vi "indexOf.vi"(8 "error in (no error)":errorcluster, 10 "Key":string, 11 "Bucket in":refnum<class "Bucket.lvclass">) -> (0 "error out":errorcluster, 2 "Index":i32, 3 "Bucket out":refnum<class "Bucket.lvclass">)   [LabVIEW 2017, in "Bucket.lvclass"]
uses:
  <userlib>/836-Library/Data_Structures/HashMap/Support/Bucket/Bucket.lvclass
  <userlib>/836-Library/Data_Structures/HashMap/Support/Bucket/Bucket.lvclass/Bucket.ctl
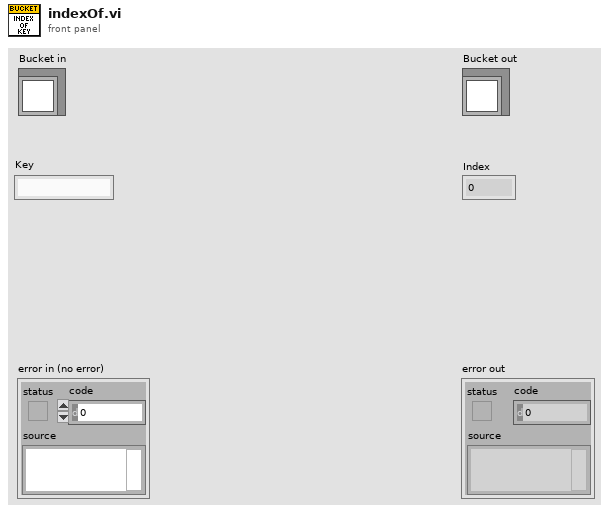
[diagram p1: front panel]
types:
  T1 = typedef "KeyValuePair.ctl" = cluster{"Key":string, "Value":variant}
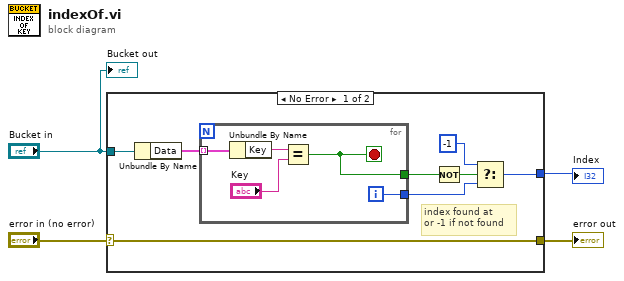
[diagram p0: block diagram]
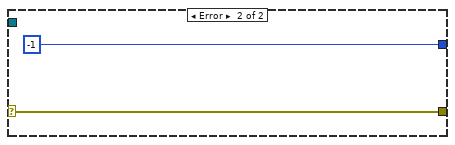
[diagram p2: hidden frame]
diagram:
  n1 = case shown="No Error" "error in (no error)" {
    selector: "error in (no error)" -> [w7 w19]
    tunnel: [w7 w19] -> w3
    tunnel: "Bucket in" -> [w6 _]
    tunnel: [w5 -1 ("t")] -> w2
    frame No Error {
      # "index found at\nor -1 if not found"
      n2 = Unbundle By Name(w6) -> ("Data"=w12:T1[])
      n3 = for {
        tunnel: w12 -> [w17] mode=indexing
        tunnel: [w14] -> w9
        tunnel: [w13] -> w11
        i -> [w14]
        stop <- w13 stop-if-true
        n4 = Unbundle By Name(w17) -> ("Key"=w16:string)
        n5 = Equal?(x=w16, y="Key") -> (x = y?=w13:bool)
      }
      n6 = Not(x=w11) -> (.not. x?=w10:bool)
      n7 = Select(t=-1, s=w10, f=w9) -> (s? t:f=w5:i32)
    }
    frame Error {
    }
  }
  "error out" <- w3
  "Index" <- w2
  "Bucket out" <- "Bucket in"
